vi "DCIR_conf_alim.vi"(8 "ErrIN":errorcluster caption="entrée d'erreur (pas d'erreur)", 11 "VISAin":refnum<visa-resource-name>) -> (0 "ErrOUT":errorcluster caption="sortie d'erreur", 3 "VisaOUT":refnum<visa-resource-name>)   [LabVIEW 2020]
uses:
  Param_Stack.vi
  <instrlib>/IT6000C/IT6000C.lvlib
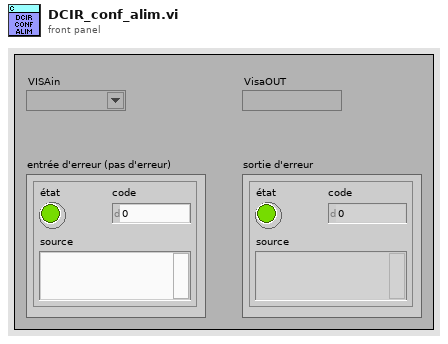
[diagram p1: front panel]
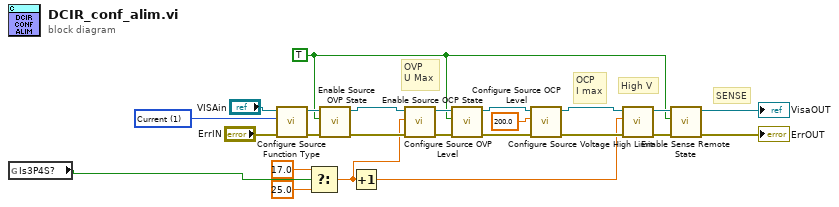
[diagram p0: block diagram]
diagram:
  w15 = u16 1 items=["Voltage", "Current"] ("Mode(0:Voltage)")
  w6 = TRUE ("Enable(True)")
  # "High V"
  # "SENSE"
  # "OVP\nU Max"
  # "OCP\nI max"
  n1 = global read "Param_Stack.vi" "Is3P4S?"() -> (w1:bool)
  n2 = call <instrlib>:"Configure Source Function Type.vi"("error in (no error)"="ErrIN", "Mode(0:Voltage)"=w15, "VISA resource name"="VISAin") -> ("error out"=w13:errorcluster, "VISA resource name out"=w14:refnum<visa-resource-name>)  [unwired: 7 in]
  n3 = Select ("Sélectionner")(t=17.0 ("cas vrai"), s=w1, f=25.0 ("cas faux")) -> (s? t:f=w2:dbl)
  n4 = call <instrlib>:"Enable Source OVP State.vi"("error in (no error)"=w13, "Enable(True)"=w6, "VISA resource name"=w14) -> ("error out"=w22:errorcluster, "VISA resource name out"=w21:refnum<visa-resource-name>)  [unwired: 7 in]
  n5 = Increment(x=w2) -> (x+1=w3:dbl)
  n6 = call <instrlib>:"Configure Source OVP Level.vi"("error in (no error)"=w22, "Value(0)"=w2, "VISA resource name"=w21) -> ("error out"=w20:errorcluster, "VISA resource name out"=w19:refnum<visa-resource-name>)  [unwired: 7 in]
  n7 = call <instrlib>:"Enable Source OCP State.vi"("error in (no error)"=w20, "Enable(True)"=w6, "VISA resource name"=w19) -> ("error out"=w17:errorcluster, "VISA resource name out"=w18:refnum<visa-resource-name>)  [unwired: 7 in]
  n8 = call <instrlib>:"Configure Source OCP Level.vi"("error in (no error)"=w17, "Value(0)"=200.0, "VISA resource name"=w18) -> ("error out"=w12:errorcluster, "VISA resource name out"=w11:refnum<visa-resource-name>)  [unwired: 7 in]
  n9 = call <instrlib>:"Configure Source Voltage High Limit.vi"("error in (no error)"=w12, "Value(0)"=w3, "VISA resource name"=w11) -> ("error out"=w10:errorcluster, "VISA resource name out"=w9:refnum<visa-resource-name>)  [unwired: 7 in]
  n10 = call <instrlib>:"Enable Sense Remote State.vi"("error in (no error)"=w10, "Enable(True)"=w6, "VISA resource name"=w9) -> ("error out"=→"ErrOUT":errorcluster, "VISA resource name out"=→"VisaOUT":refnum<visa-resource-name>)  [unwired: 7 in]
